vi "Trav_pos_global.vi"() -> ()   [LabVIEW 2015]
uses:
  Gen Trav/Traverse_cluster.ctl
  Gen Trav/Spacing.ctl
  Controls/Multi_run_mode.ctl
  Controls/Tunnel_Coordinates.ctl
panel:
  out "Trav Last Moved":timestamp
  in  "Current Image Filename":path
  in  "Sync to server now":bool
  in  "Traverses to Move":string[](array[string])
  in  "Traverse Origin X Offset (mm)":sgl min=0 max=20000
  in  "Traverse Output Board Number":u32=1
  in  "Traverse Computer IP Number":string
  in  "Live Position":sgl[](array[numeric])=[0.0, 0.0, 0.0] format="%.6f"
  in  "ADAM Positions Ch names":string[](array[string])
  in  "Route checking Chs":string[](array[string])
  in  "Pause Until Seconds 1904":dbl
  in  "FFID Background":T1 {"Carrier_2 Q (l/min)" format="%#.2f"; "Row Duration (mins)" format="%#.1f"; "Row No" min=0; "Trace Gas Concentration (%)" min=0.0 format="%#_4f"; "Carrier_1 Q (l/min)" format="%#.2f"; "Tunnel Speed" format="%#.2f"; "Start X" format="%#.2f"; "Start Y" format="%#.2f"; "Start Z" format="%#.2f"; "End X" format="%#.2f"; "End Y" format="%#.2f"; "End Z" format="%#.2f"; "Averaging time (min)" min=0.0 format="%#.2f"}
  in  "Meas Setup Number":i32
  in  "Current Meas Setup File":string
  in  "Default Traverse Setup":string
  out "Simulation Time":timestamp
  out "Row completion times":timestamp[](array[timestamp])
  in  "Dummy Measurement?":bool
  in  "Jumped Positions":dbl[][](array[numeric])
  in  "Jump Bad Positions?":bool
  in  "Work in Tunnel Coordinates?":T4
  in  "Show User Metadata on Launch?":bool=TRUE
  in  "Measurement setup files":string[](array[string])
  out "Live Traverse Preview?":bool
  in  "Paused During Row?":bool
  in  "Speed Factor":sgl=1.0 min=0.1 max=60 format="%.2f"
  in  "Estimated Completion time":string
  in  "Start of Row time (Sec)":dbl
  out "Currently on point":i32=9
  in  "Current Row":T1 {"Carrier_2 Q (l/min)" format="%#.2f"; "Row Duration (mins)" format="%#.1f"; "Row No" min=0; "Trace Gas Concentration (%)" min=0.0 format="%#_4f"; "Carrier_1 Q (l/min)" format="%#.2f"; "Tunnel Speed" format="%#.2f"; "Start X" format="%#.2f"; "Start Y" format="%#.2f"; "Start Z" format="%#.2f"; "End X" format="%#.2f"; "End Y" format="%#.2f"; "End Z" format="%#.2f"; "Averaging time (min)" min=0.0 format="%#.2f"}
  in  "Source Control?":bool
  in  "Top level setup filename":path
  in  "Pause Acquisition":bool
  out "Axis Traversed":enum16{"X traverse", "Y traverse", "Z traverse"}(ring)
  in  "Traverse position":sgl[](array[numeric])=[0.0, 0.0, 0.0] format="%.2f"
  # "X                Y                   Z"
  # "X           Y            Z"
  # "Start"
  # "End"
  # "X           Y            Z"
  # "Start"
  # "End"
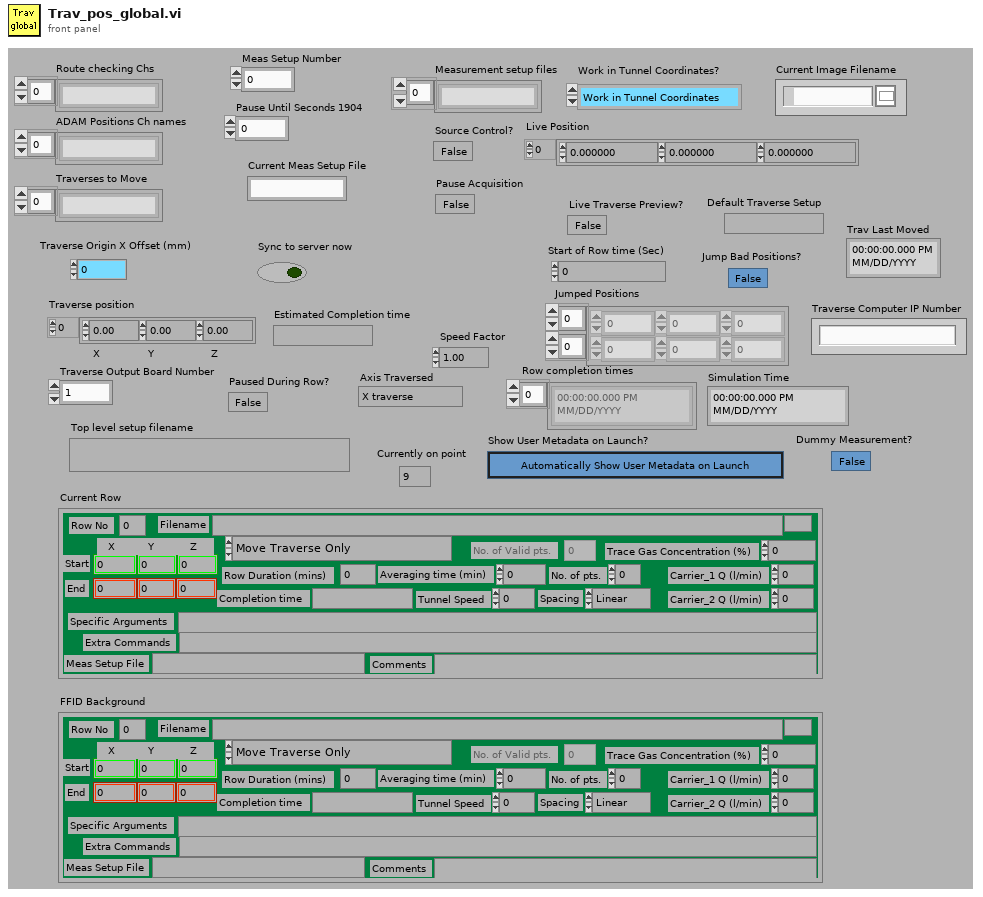
[diagram p1: front panel]
types:
  T1 = typedef "Traverse_cluster.ctl" = cluster{"Start X":sgl, "Start Y":sgl, "Start Z":sgl, "End X":sgl, "End Y":sgl, "End Z":sgl, "No. of pts.":i32, "Spacing":T2, "Filename":path, "Tunnel Speed":dbl, "Averaging time (min)":dbl, "Extra Commands":string, "Carrier_1 Q (l/min)":dbl, "Carrier_2 Q (l/min)":dbl, "Trace Gas Concentration (%)":dbl, "Specific Arguments":string, "Comments":string, "Row No":i32, "Row Type Selector":T3, "Completion time":string, "Row Duration (mins)":dbl, "No. of Valid pts.":i32, "Meas Setup File":string}
  T2 = typedef "Spacing.ctl" = enum16{"Linear", "Log", "Gauss", "Specified", "N/A"}
  T3 = typedef "Multi_run_mode.ctl" = enum16{"Move Traverse Only", "Set Tunnel Speed Only", "Set Source Only", "Set Measurement Conditions", "Single Measurement", "Vertical Profile", "Lateral Profile", "Longitudinal Profile", "Explore Volume", "Multi-Axis Profile", "Auto Calibrate", "Meas Fast FID Bkgnd", "Check Beam Power", "Scanning Valve Measurement", "Run VI Named:", "Set ADAM Ch", "Wait (minutes)", "Send Message", "Synchronize With:", "Fall Back to this Row", "Turn Off Row Repeating", "Blank Row", "Traverse 3D Volume"}
  T4 = typedef "Tunnel_Coordinates.ctl" = enum16{"Work in Tunnel Coordinates", "Work in Model Coordinates"}
diagram:
